vi "Generate Hawkeye File.vi"(6 "Regenerate?":bool, 7 "Status Indicator Ref":refnum<vi>, 8 "error in (no error)":errorcluster, 9 "Check Changed Libraries Only?":bool, 10 "LVLib / LVClass / Sub Folder Path":path, 11 "Repo Folder Path":path=path "C:/sw-deps-monitor/Source/BuildSpecs") -> (0 "error out":errorcluster)   [LabVIEW 2019, in "Hawkeye.lvlib"]
uses:
  Hawkeye.lvlib
  <userlib>/_OpenG.lib/file/file.llb/File Exists - Scalar__ogtk.vi
  <userlib>/_OpenG.lib/file/file.llb/Compare Two Paths - Scalar__ogtk.vi
  <vilib>/Utility/config.llb/NI_LVConfig.lvlib
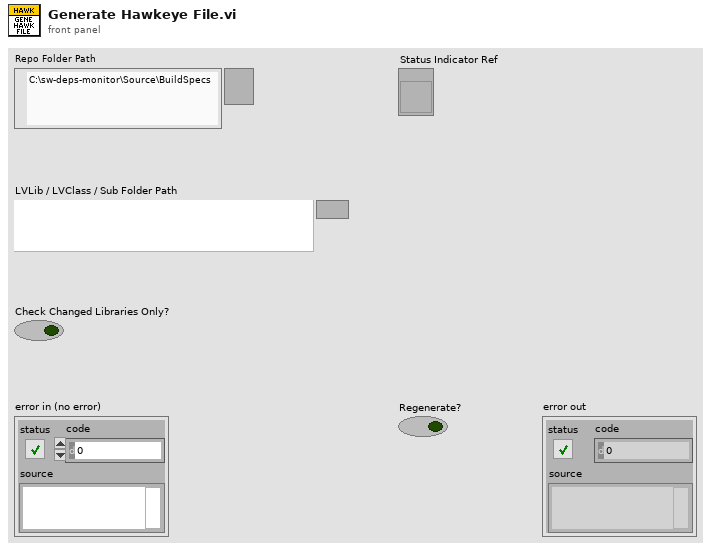
[diagram p1: front panel]
types:
  T1 = typedef "NI_LVConfig.lvlib/Config Data RefNum.ctl" = refnum<k1>
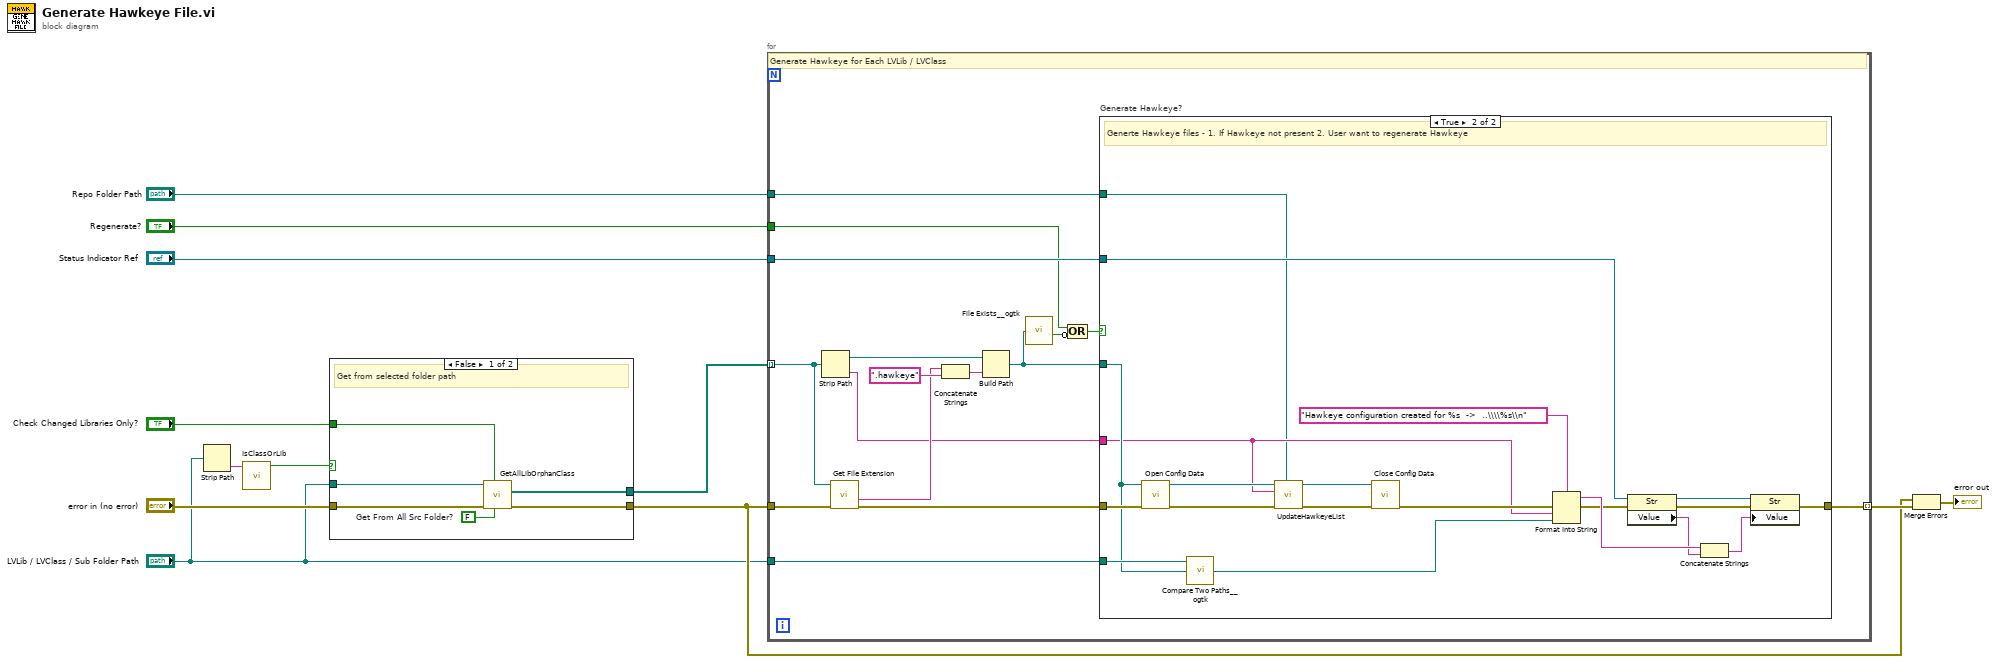
[diagram p0: block diagram]
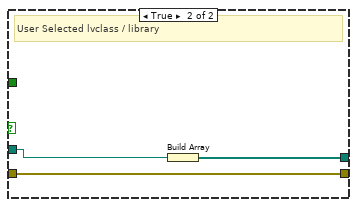
[diagram p2: hidden frame]
diagram:
  n1 = Strip Path(path="LVLib / LVClass / Sub Folder Path") -> (name=w7:string)  [unwired: 1 out]
  n2 = call "IsClassOrLib.vi"("LVFile Name"=w7) -> ("Is LVClass or Library?"=w4:bool)  [unwired: 10 in]
  n3 = case shown="False" w4 {
    tunnel: "error in (no error)" -> [w18 w20]
    tunnel: [w17 w20] -> w5
    tunnel: "Check Changed Libraries Only?" -> [w16 _]
    tunnel: [w15 w19] -> w2
    tunnel: "LVLib / LVClass / Sub Folder Path" -> [w14 w21]
    frame False {
      w13 = FALSE  # Get From All Src Folder?
      # "Get from selected folder path"
      n4 = call "GetAllLibOrphanClass.vi"("Get From All Src Folder?"=w13, "ListForChangedLibrariesOnly"=w16, "error in (no error)"=w18, "Workspace Path"=w14) -> ("error out"=w17:errorcluster, "Lib / Class Path []"=w15:path[])  [unwired: 5 in, 1 out]
    }
    frame True {
      # "User Selected lvclass / library"
      n5 = Build Array(w21) -> (w19:path[])
    }
  }
  n6 = for {
    tunnel: "Status Indicator Ref" -> [w37]
    tunnel: w2 -> [w29] mode=indexing
    tunnel: w5 -> [w33]
    tunnel: "LVLib / LVClass / Sub Folder Path" -> [w32]
    tunnel: [w31] -> w12 mode=indexing
    tunnel: "Regenerate?" -> [w23]
    tunnel: "Repo Folder Path" -> [w22]
    # "Generate Hawkeye for Each LVLib / LVClass"
    n7 = Strip Path(path=w29) -> (stripped path=w30:path, name=w27:string)
    n8 = call <vilib>:"Get File Extension.vi"("error in (no error)"=w33, "file"=w29) -> ("error out"=w36:errorcluster, "filename without extension"=w28:string)  [unwired: 5 in, 3 out]
    n9 = Concatenate Strings(w28, ".hawkeye" ("string")) -> (w35:string)
    n10 = Build Path(base path=w30, name or relative path=w35) -> (appended path=w26:path)
    n11 = call-poly <userlib>:"File Exists__ogtk.vi"("file path"=w26) -> ("exists"=w25:bool)  [unwired: 6 in, 1 out]
    n12 = Compound Arithmetic op=OR(w23, invert w25) -> (w24:bool)
    n13 = case "Generate Hawkeye?" shown="True" w24 {
      tunnel: w37 -> [_ w58]
      tunnel: w36 -> [w38 w57]
      tunnel: w32 -> [_ w48]
      tunnel: [w38 w46] -> w31
      tunnel: w26 -> [_ w45]
      tunnel: w27 -> [_ w40]
      tunnel: w22 -> [_ w39]
      frame False {
      }
      frame True {
        # "Generte Hawkeye files - 1. If Hawkeye not present 2. User want to regenerate Hawkeye"
        n14 = call <vilib>:"Open Config Data.vi"("error in (no error)"=w57, "configuration file path"=w45) -> ("error out"=w42:errorcluster, "refnum"=w43:T1)  [unwired: 7 in, 1 out]
        n15 = call-poly <userlib>:"Compare Two Paths__ogtk.vi"("path2"=w45, "path1"=w48) -> ("relative path from 1 to 2"=w51:path)  [unwired: 1 in, 2 out]
        n16 = call "UpdateHawkeyeList.vi"("WorkSpace / Repo path"=w39, "error in (no error)"=w42, "Library/Class Name"=w40, "Config Refnum in"=w43) -> ("error out"=w41:errorcluster, "Config Refnum out"=w44:T1)  [unwired: 4 in, 2 out]
        n17 = call <vilib>:"Close Config Data.vi"("error in (no error)"=w41, "refnum"=w44) -> ("error out"=w50:errorcluster)  [unwired: 8 in, 1 out]
        n18 = Format Into String(format string="Hawkeye configuration created for %s  ->  ..\\\\%s\\n", error in=w50, w40, w51) -> (resulting string=w52:string, error out=w49:errorcluster)  [unwired: 1 in]
        n19 = property on="Property Node" class="Str"(reference=w58, error in=w49) -> (reference out=w54:refnum<vi>, error out=w53:errorcluster, "Value"=w47:string)
        n20 = Concatenate Strings(w52, w47) -> (w55:string)
        n21 = property on="Property Node" class="Str"(reference=w54, error in=w53, "Value"=w55) -> (error out=w46:errorcluster)  [unwired: 1 out]
      }
    }
  }
  n22 = Merge Errors(w5, w12) -> (→"error out":errorcluster)
